vi "ScaleBias.vi"(9 "Waveform in":waveform(dbl), 10 "Bias":dbl, 11 "Scale":dbl) -> (3 "Waveform out":waveform(dbl))   [LabVIEW 2013]
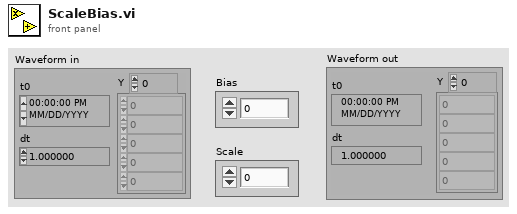
[diagram p1: front panel]
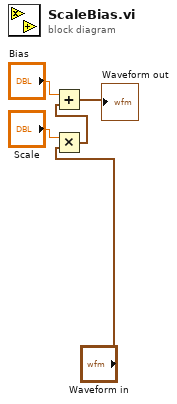
[diagram p0: block diagram]
diagram:
  n1 = Multiply(x="Scale", y="Waveform in") -> (x*y=w2:waveform(dbl))
  n2 = Add(x="Bias", y=w2) -> (x+y=→"Waveform out":waveform(dbl))
